vi "debugging project symbols.vi"() -> ()   [LabVIEW 2020]
panel:
  in  "Nominal Debug Symbols":cluster{"String":string, "Boolean":bool}[](array[cluster])
  # "I probably wouldn't recommend using this tool.\nIf you have any other symbols, this will remove them."
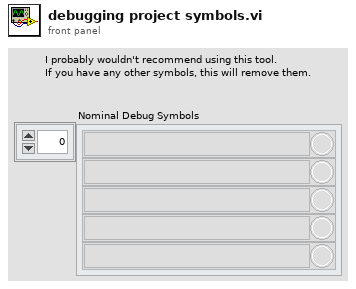
[diagram p1: front panel]
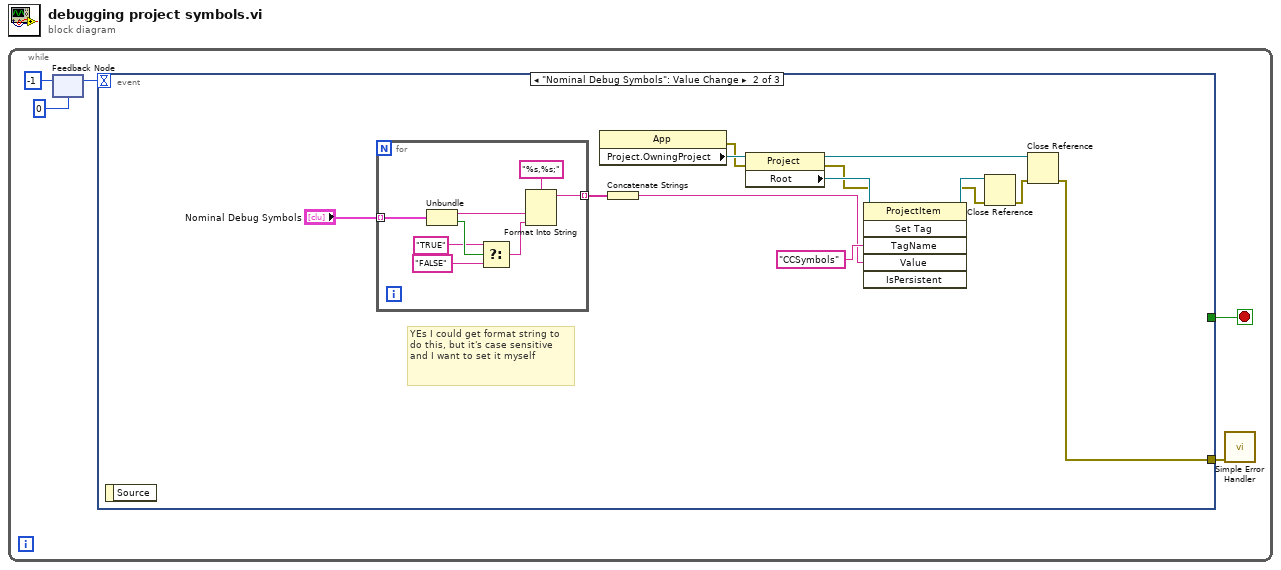
[diagram p0: block diagram]
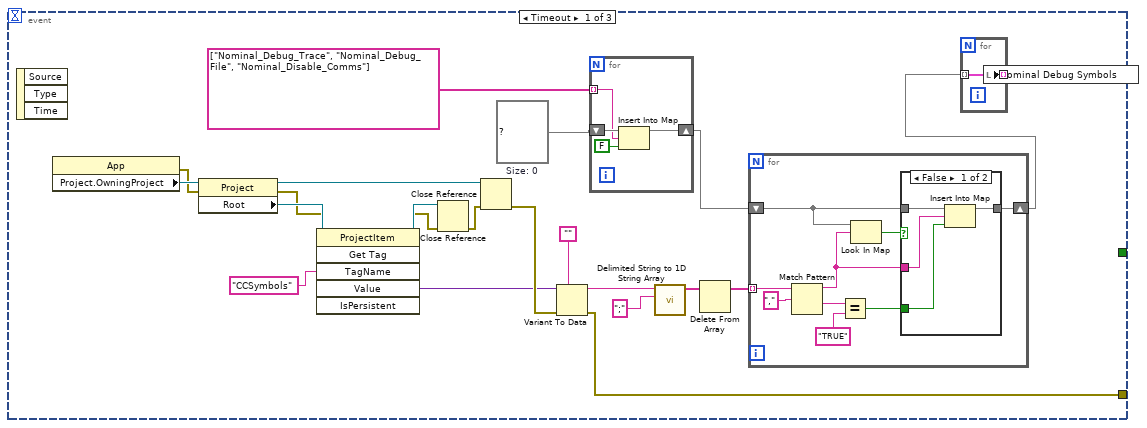
[diagram p2: hidden frame]
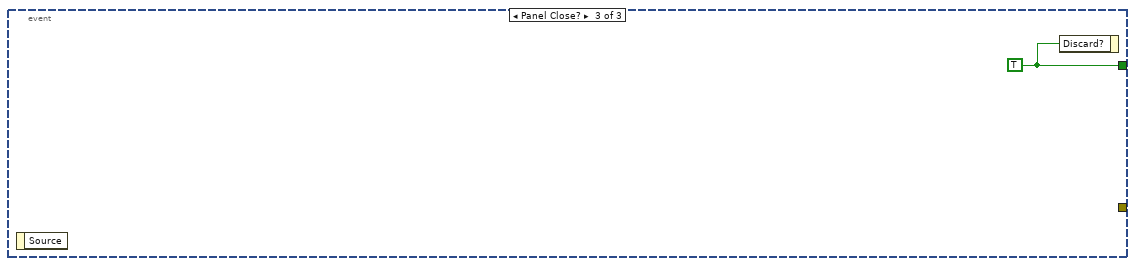
[diagram p4: hidden frame]
diagram:
  n1 = while {
    stop <- w2 stop-if-true
    n2 = feedback-in #1(-1) -> ()
    n3 = feedback #1(0) -> (w4:i32)
    n4 = event shown="[1] \"Nominal Debug Symbols\": Value Change" {
      selector: _ -> [_ _ _]
      dyn-events: _ -> [_ _ _]
      timeout: w4 -> [_ _ _]
      tunnel: [_ _ w68] -> w2
      tunnel: [w6 w47 _] -> w1
      event Timeout {
        w11 = map{string, bool} {}  # Size: 0
        n5 = event-data() -> ()  [unwired: 1 in, 3 out]
        n6 = property class="App"() -> (error out=w19:errorcluster, "Project.OwningProject"=w26:refnum<vi>)  [unwired: 2 in, 1 out]
        n7 = property class="Project"(reference=w26, error in=w19) -> (reference out=w17:refnum<vi>, error out=w20:errorcluster, "Root"=w25:refnum<vi>)
        n8 = invoke class="ProjectItem" method="Get Tag"(reference=w25, error in=w20, "TagName"="CCSymbols" ("Tag Name")) -> (reference out=w23:refnum<vi>, error out=w18:errorcluster, "Value"=w22:variant)  [unwired: 3 in, 3 out]
        n9 = Close Reference(reference=w23, error in (no error)=w18) -> (error out=w16:errorcluster)
        n10 = Close Reference(reference=w17, error in (no error)=w16) -> (error out=w27:errorcluster)
        n11 = Variant To Data(error in=w27, type="", Variant=w22) -> (data=w14:string, error out=w6:errorcluster)
        n12 = for {
          shift-right: [w30] -> w9
          shift-left: w11 -> [w32]
          tunnel: string[] ["Nominal_Debug_Trace", "Nominal_Debug_File", "Nominal_Disable_Comms"] -> [w31] mode=indexing
          n13 = Insert Into Map(map in=w32, key=w31, value=FALSE) -> (map out=w30:map{string, bool})  [unwired: 2 out]
        }
        n14 = call <vilib>:"Delimited String to 1D String Array.vi"("delimiter"=";", "delimited string"=w14) -> ("string array"=w13:string[])  [unwired: 9 in]
        n15 = Delete From Array(array=w13) -> (array with subset deleted=w12:string[])  [unwired: 2 in, 1 out]
        n16 = for {
          tunnel: w12 -> [w40] mode=indexing
          shift-right: [w36] -> w8
          shift-left: w9 -> [w35]
          n17 = Match Pattern(string=w40, regular expression=",") -> (before substring=w34:string, after substring=w39:string)  [unwired: 1 in, 2 out]
          n18 = Equal?(x=w39, y="TRUE") -> (x = y?=w33:bool)
          n19 = Look In Map(map=w35, key=w34) -> (key not found?=w37:bool)  [unwired: 1 in, 1 out]
          n20 = case shown="False" w37 {
            tunnel: [w42 w46] -> w36
            tunnel: w35 -> [w45 w46]
            tunnel: w34 -> [w44 _]
            tunnel: w33 -> [w43 _]
            frame False {
              n21 = Insert Into Map(map in=w45, key=w44, value=w43) -> (map out=w42:map{string, bool})  [unwired: 2 out]
            }
            frame True {
            }
          }
        }
        n22 = for {
          tunnel: w8 -> [w28] mode=indexing
          tunnel: [w28] -> w7 mode=indexing
        }
        n23 = local write "Nominal Debug Symbols"(w7) -> ()
      }
      event "Nominal Debug Symbols": Value Change {
        # "YEs I could get format string to do this, but it's case sensitive and I want to set it myself"
        n24 = event-data() -> ()  [unwired: 1 in, 1 out]
        n25 = for {
          tunnel: "Nominal Debug Symbols" -> [w67] mode=indexing
          tunnel: [w60] -> w58 mode=indexing
          n26 = Unbundle(w67) -> ("String"=w61:string, "Boolean"=w66:bool)
          n27 = Select(t="TRUE", s=w66, f="FALSE") -> (s? t:f=w62:string)
          n28 = Format Into String(format string="%s,%s;", w61, w62) -> (resulting string=w60:string)  [unwired: 2 in, 1 out]
        }
        n29 = property class="App"() -> (error out=w52:errorcluster, "Project.OwningProject"=w57:refnum<vi>)  [unwired: 2 in, 1 out]
        n30 = Concatenate Strings(w58) -> (w48:string)
        n31 = property class="Project"(reference=w57, error in=w52) -> (reference out=w50:refnum<vi>, error out=w53:errorcluster, "Root"=w56:refnum<vi>)
        n32 = invoke class="ProjectItem" method="Set Tag"(reference=w56, error in=w53, "TagName"="CCSymbols" ("Tag Name"), "Value"=w48) -> (reference out=w54:refnum<vi>, error out=w51:errorcluster)  [unwired: 2 in, 4 out]
        n33 = Close Reference(reference=w54, error in (no error)=w51) -> (error out=w49:errorcluster)
        n34 = Close Reference(reference=w50, error in (no error)=w49) -> (error out=w47:errorcluster)
      }
      event Panel Close? {
        w68 = TRUE
        n35 = event-data() -> ()  [unwired: 1 in, 1 out]
        n36 = event-data("Discard?"=w68) -> ()  [unwired: 1 in, 1 out]
      }
    }
    n37 = call <vilib>:"Simple Error Handler.vi"("error in (no error)"=w1) -> ()  [unwired: 4 in, 5 out]
  }
